vi "salMain.vi"() -> ()   [LabVIEW 2012]
uses:
  TypeConstructor/TypeConstructor.lvclass
  Typedefs/ElementType.ctl
panel:
  out "error out":errorcluster
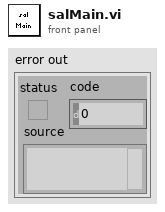
[diagram p1: front panel]
types:
  T1 = typedef "ElementType.ctl" = enum16{"string", "double", "long", "short", "long long", "unsigned short", "unsigned long", "unsigned long long", "float", "char", "boolean", "short array", "long array", "long long array", "unsigned short array", "unsigned long array", "unsigned long long array", "float array", "double array", "char array", "boolean array"}
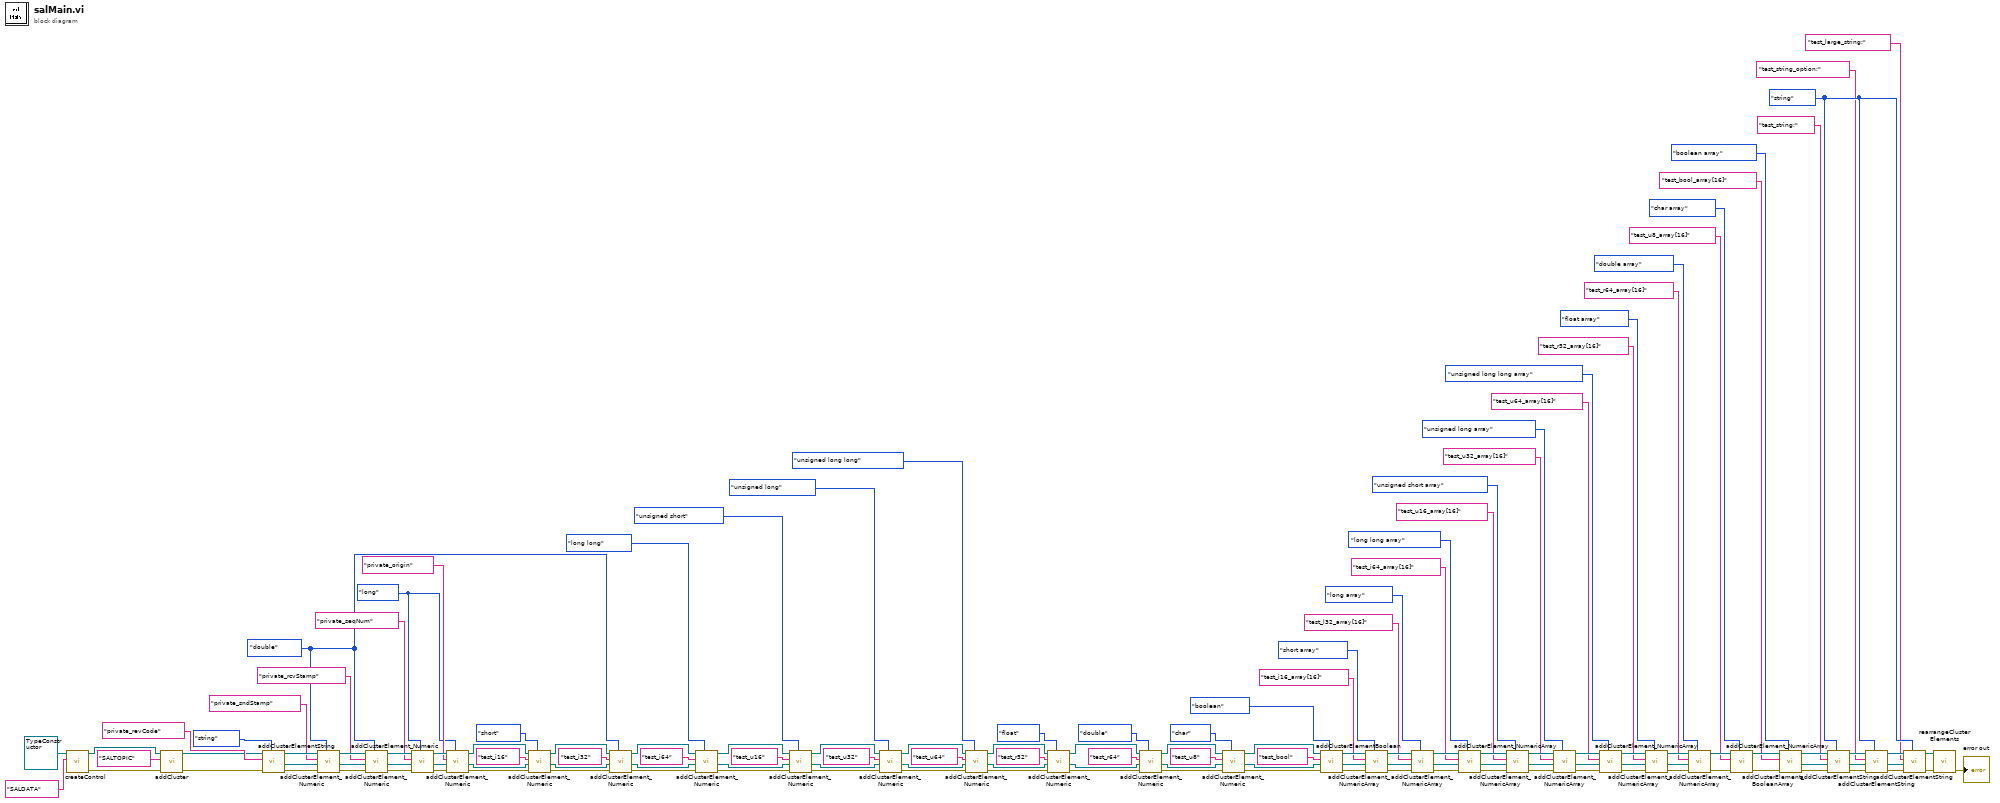
[diagram p0: block diagram]
diagram:
  w4 = ElementType."string" ("ElementType")
  w114 = ElementType."long" ("ElementType")
  w104 = ElementType."double" ("ElementType")
  n1 = call "createControl.vi"("name"="SALDATA", "TypeConstructor in"=refnum<class "TypeConstructor.lvclass"> refnum) -> ("error out"=w137:errorcluster, "TypeConstructor out"=w139:refnum<class "TypeConstructor.lvclass">)  [unwired: 8 in]
  n2 = call "addCluster.vi"("error in (no error)"=w137, "name"="SALTOPIC", "TypeConstructor in"=w139) -> ("error out"=w135:errorcluster, "TypeConstructor out"=w133:refnum<class "TypeConstructor.lvclass">)  [unwired: 7 in]
  n3 = call "addClusterElementString.vi"("ElementType"=ElementType."string", "error in (no error)"=w135, "name"="private_revCode", "TypeConstructor in"=w133) -> ("error out"=w131:errorcluster, "thisControlRef"=w130:refnum<vi>, "TypeConstructor out"=w129:refnum<class "TypeConstructor.lvclass">)  [unwired: 5 in]
  n4 = call "addClusterElement_Numeric.vi"("ElementType"=w104, "error in (no error)"=w131, "prevObjRef"=w130, "name"="private_sndStamp", "TypeConstructor in"=w129) -> ("error out"=w125:errorcluster, "thisControlRef"=w124:refnum<vi>, "TypeConstructor out"=w126:refnum<class "TypeConstructor.lvclass">)  [unwired: 4 in]
  n5 = call "addClusterElement_Numeric.vi"("ElementType"=w104, "error in (no error)"=w125, "prevObjRef"=w124, "name"="private_rcvStamp", "TypeConstructor in"=w126) -> ("error out"=w122:errorcluster, "thisControlRef"=w121:refnum<vi>, "TypeConstructor out"=w120:refnum<class "TypeConstructor.lvclass">)  [unwired: 4 in]
  n6 = call "addClusterElement_Numeric.vi"("ElementType"=w114, "error in (no error)"=w122, "prevObjRef"=w121, "name"="private_seqNum", "TypeConstructor in"=w120) -> ("error out"=w118:errorcluster, "thisControlRef"=w117:refnum<vi>, "TypeConstructor out"=w116:refnum<class "TypeConstructor.lvclass">)  [unwired: 4 in]
  n7 = call "addClusterElement_Numeric.vi"("ElementType"=w114, "error in (no error)"=w118, "prevObjRef"=w117, "name"="private_origin", "TypeConstructor in"=w116) -> ("error out"=w113:errorcluster, "thisControlRef"=w112:refnum<vi>, "TypeConstructor out"=w111:refnum<class "TypeConstructor.lvclass">)  [unwired: 4 in]
  n8 = call "addClusterElement_Numeric.vi"("ElementType"=ElementType."short", "error in (no error)"=w113, "prevObjRef"=w112, "name"="test_i16", "TypeConstructor in"=w111) -> ("error out"=w108:errorcluster, "thisControlRef"=w107:refnum<vi>, "TypeConstructor out"=w106:refnum<class "TypeConstructor.lvclass">)  [unwired: 4 in]
  n9 = call "addClusterElement_Numeric.vi"("ElementType"=w104, "error in (no error)"=w108, "prevObjRef"=w107, "name"="test_i32", "TypeConstructor in"=w106) -> ("error out"=w103:errorcluster, "thisControlRef"=w102:refnum<vi>, "TypeConstructor out"=w101:refnum<class "TypeConstructor.lvclass">)  [unwired: 4 in]
  n10 = call "addClusterElement_Numeric.vi"("ElementType"=ElementType."long long", "error in (no error)"=w103, "prevObjRef"=w102, "name"="test_i64", "TypeConstructor in"=w101) -> ("error out"=w98:errorcluster, "thisControlRef"=w97:refnum<vi>, "TypeConstructor out"=w96:refnum<class "TypeConstructor.lvclass">)  [unwired: 4 in]
  n11 = call "addClusterElement_Numeric.vi"("ElementType"=ElementType."unsigned short", "error in (no error)"=w98, "prevObjRef"=w97, "name"="test_u16", "TypeConstructor in"=w96) -> ("error out"=w95:errorcluster, "thisControlRef"=w94:refnum<vi>, "TypeConstructor out"=w93:refnum<class "TypeConstructor.lvclass">)  [unwired: 4 in]
  n12 = call "addClusterElement_Numeric.vi"("ElementType"=ElementType."unsigned long", "error in (no error)"=w95, "prevObjRef"=w94, "name"="test_u32", "TypeConstructor in"=w93) -> ("error out"=w92:errorcluster, "thisControlRef"=w91:refnum<vi>, "TypeConstructor out"=w90:refnum<class "TypeConstructor.lvclass">)  [unwired: 4 in]
  n13 = call "addClusterElement_Numeric.vi"("ElementType"=ElementType."unsigned long long", "error in (no error)"=w92, "prevObjRef"=w91, "name"="test_u64", "TypeConstructor in"=w90) -> ("error out"=w80:errorcluster, "thisControlRef"=w79:refnum<vi>, "TypeConstructor out"=w81:refnum<class "TypeConstructor.lvclass">)  [unwired: 4 in]
  n14 = call "addClusterElement_Numeric.vi"("ElementType"=ElementType."float", "error in (no error)"=w80, "prevObjRef"=w79, "name"="test_r32", "TypeConstructor in"=w81) -> ("error out"=w82:errorcluster, "thisControlRef"=w83:refnum<vi>, "TypeConstructor out"=w78:refnum<class "TypeConstructor.lvclass">)  [unwired: 4 in]
  n15 = call "addClusterElement_Numeric.vi"("ElementType"=ElementType."double", "error in (no error)"=w82, "prevObjRef"=w83, "name"="test_r64", "TypeConstructor in"=w78) -> ("error out"=w73:errorcluster, "thisControlRef"=w72:refnum<vi>, "TypeConstructor out"=w71:refnum<class "TypeConstructor.lvclass">)  [unwired: 4 in]
  n16 = call "addClusterElement_Numeric.vi"("ElementType"=ElementType."char", "error in (no error)"=w73, "prevObjRef"=w72, "name"="test_u8", "TypeConstructor in"=w71) -> ("error out"=w68:errorcluster, "thisControlRef"=w67:refnum<vi>, "TypeConstructor out"=w66:refnum<class "TypeConstructor.lvclass">)  [unwired: 4 in]
  n17 = call "addClusterElementBoolean.vi"("ElementType"=ElementType."boolean", "error in (no error)"=w68, "prevObjRef"=w67, "name"="test_bool", "TypeConstructor in"=w66) -> ("error out"=w59:errorcluster, "thisControlRef"=w60:refnum<vi>, "TypeConstructor out"=w63:refnum<class "TypeConstructor.lvclass">)  [unwired: 4 in]
  n18 = call "addClusterElement_NumericArray.vi"("ElementType"=ElementType."short array", "error in (no error)"=w59, "prevObjRef"=w60, "name"="test_i16_array[16]", "TypeConstructor in"=w63) -> ("error out"=w58:errorcluster, "thisControlRef"=w57:refnum<vi>, "TypeConstructor out"=w56:refnum<class "TypeConstructor.lvclass">)  [unwired: 4 in]
  n19 = call "addClusterElement_NumericArray.vi"("ElementType"=ElementType."long array", "error in (no error)"=w58, "prevObjRef"=w57, "name"="test_l32_array[16]", "TypeConstructor in"=w56) -> ("error out"=w53:errorcluster, "thisControlRef"=w52:refnum<vi>, "TypeConstructor out"=w51:refnum<class "TypeConstructor.lvclass">)  [unwired: 4 in]
  n20 = call "addClusterElement_NumericArray.vi"("ElementType"=ElementType."long long array", "error in (no error)"=w53, "prevObjRef"=w52, "name"="test_i64_array[16]", "TypeConstructor in"=w51) -> ("error out"=w48:errorcluster, "thisControlRef"=w47:refnum<vi>, "TypeConstructor out"=w46:refnum<class "TypeConstructor.lvclass">)  [unwired: 4 in]
  n21 = call "addClusterElement_NumericArray.vi"("ElementType"=ElementType."unsigned short array", "error in (no error)"=w48, "prevObjRef"=w47, "name"="test_u16_array[16]", "TypeConstructor in"=w46) -> ("error out"=w43:errorcluster, "thisControlRef"=w42:refnum<vi>, "TypeConstructor out"=w41:refnum<class "TypeConstructor.lvclass">)  [unwired: 4 in]
  n22 = call "addClusterElement_NumericArray.vi"("ElementType"=ElementType."unsigned long array", "error in (no error)"=w43, "prevObjRef"=w42, "name"="test_u32_array[16]", "TypeConstructor in"=w41) -> ("error out"=w38:errorcluster, "thisControlRef"=w37:refnum<vi>, "TypeConstructor out"=w36:refnum<class "TypeConstructor.lvclass">)  [unwired: 4 in]
  n23 = call "addClusterElement_NumericArray.vi"("ElementType"=ElementType."unsigned long long array", "error in (no error)"=w38, "prevObjRef"=w37, "name"="test_u64_array[16]", "TypeConstructor in"=w36) -> ("error out"=w33:errorcluster, "thisControlRef"=w32:refnum<vi>, "TypeConstructor out"=w31:refnum<class "TypeConstructor.lvclass">)  [unwired: 4 in]
  n24 = call "addClusterElement_NumericArray.vi"("ElementType"=ElementType."float array", "error in (no error)"=w33, "prevObjRef"=w32, "name"="test_r32_array[16]", "TypeConstructor in"=w31) -> ("error out"=w28:errorcluster, "thisControlRef"=w27:refnum<vi>, "TypeConstructor out"=w26:refnum<class "TypeConstructor.lvclass">)  [unwired: 4 in]
  n25 = call "addClusterElement_NumericArray.vi"("ElementType"=ElementType."double array", "error in (no error)"=w28, "prevObjRef"=w27, "name"="test_r64_array[16]", "TypeConstructor in"=w26) -> ("error out"=w22:errorcluster, "TypeConstructor out"=w23:refnum<class "TypeConstructor.lvclass">)  [unwired: 4 in, 1 out]
  n26 = call "addClusterElement_NumericArray.vi"("ElementType"=ElementType."char array", "error in (no error)"=w22, "name"="test_u8_array[16]", "TypeConstructor in"=w23) -> ("error out"=w18:errorcluster, "TypeConstructor out"=w19:refnum<class "TypeConstructor.lvclass">)  [unwired: 5 in, 1 out]
  n27 = call "addClusterElement_BooleanArray.vi"("ElementType"=ElementType."boolean array", "error in (no error)"=w18, "name"="test_bool_array[16]", "TypeConstructor in"=w19) -> ("error out"=w12:errorcluster, "thisControlRef"=w11:refnum<vi>, "TypeConstructor out"=w13:refnum<class "TypeConstructor.lvclass">)  [unwired: 5 in]
  n28 = call "addClusterElementString.vi"("ElementType"=w4, "error in (no error)"=w12, "prevObjRef"=w11, "name"="test_string;", "TypeConstructor in"=w13) -> ("error out"=w16:errorcluster, "thisControlRef"=w15:refnum<vi>, "TypeConstructor out"=w14:refnum<class "TypeConstructor.lvclass">)  [unwired: 4 in]
  n29 = call "addClusterElementString.vi"("ElementType"=w4, "error in (no error)"=w16, "prevObjRef"=w15, "name"="test_string_option;", "TypeConstructor in"=w14) -> ("error out"=w10:errorcluster, "thisControlRef"=w9:refnum<vi>, "TypeConstructor out"=w8:refnum<class "TypeConstructor.lvclass">)  [unwired: 4 in]
  n30 = call "addClusterElementString.vi"("ElementType"=w4, "error in (no error)"=w10, "prevObjRef"=w9, "name"="test_large_string;", "TypeConstructor in"=w8) -> ("error out"=w6:errorcluster, "TypeConstructor out"=w7:refnum<class "TypeConstructor.lvclass">)  [unwired: 4 in, 1 out]
  n31 = call "rearrangeClusterElements.vi"("error in (no error)"=w6, "TypeConstructor in"=w7) -> ("error out"=→"error out":errorcluster)  [unwired: 8 in, 1 out]
